vi "20TDewar_Set_Heater_Value.vi"(8 "error in (no error)":errorcluster, 10 "20T-Dewar-Cluster":T1={"Dewar Heater (%)"=0.0, "D-Heater (%) Display"=3.4572, "D-Heater SP"=0.0, "Set D-Heater SP"=FALSE, "Change D-Heater Status"=FALSE, "Dewar Pressure"=0.0, "Dewar heater manual"=FALSE} {"Dewar Pressure" format="%4_5f"; "D-Heater (%) Display" format="%4_5f"; "Dewar Heater (%)" scale=0.0..100.0}, 11 "Mercury Reference In":T2) -> (0 "error out":errorcluster)   [LabVIEW 2016]
uses:
  Equipment/Mercury iXX/Public/Controls/Mercury Reference.ctl
  Equipment/Mercury iXX/Public/Controls/Comms Transport Layer.ctl
  Equipment/Mercury iXX/Private/Controls/Query Dynamic Reference.ctl
  Utility/Monitor Communication/Gustav/20T_Dewar_Cluster.ctl
  Equipment/Mercury iXX/Public/Libraries/Pressure/Open/Open Pressure Device.vi
  Equipment/Mercury iXX/Mercury iXX.lvlib
  Equipment/Mercury iXX/Public/Libraries/Pressure.lvlib
  Equipment/Mercury iXX/Public/Libraries/Control Loop.lvlib
panel:
  # "Dewar Heater (%)"
  # "Dewar Pressure"
  # "Setpoint"
  # "20T Dewar"
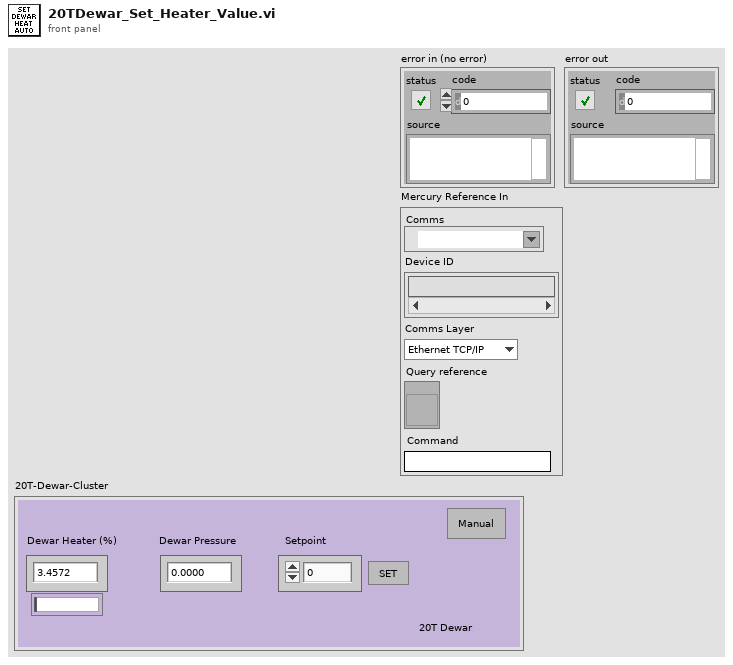
[diagram p1: front panel]
types:
  T1 = typedef "20T_Dewar_Cluster.ctl" = cluster{"Dewar Heater (%)":dbl, "D-Heater (%) Display":dbl, "D-Heater SP":dbl, "Set D-Heater SP":bool, "Change D-Heater Status":bool, "Dewar Pressure":dbl, "Dewar heater manual":bool}
  T2 = typedef "Mercury iXX.lvlib/Mercury Reference.ctl" = cluster{"Comms":refnum<visa-resource-name>, "Device ID":string[], "Comms Layer":T3, "Command":string, "Query reference":T4}
  T3 = typedef "Mercury iXX.lvlib/Comms Transport Layer.ctl" = enum16{"Ethernet TCP/IP", "USB", "ISOBus - RS-232", "GPIB"}
  T4 = typedef "Mercury iXX.lvlib/Query Dynamic Reference.ctl" = refnum<vi>
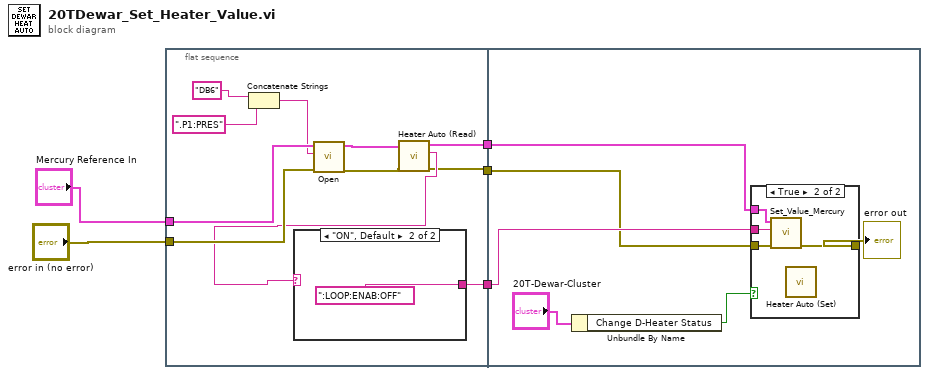
[diagram p0: block diagram]
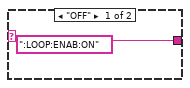
[diagram p2: hidden frame]
diagram:
  n1 = flat-sequence {
    tunnel: "Mercury Reference In" -> [w16]
    tunnel: "error in (no error)" -> [w15]
    tunnel: [w6] -> w3
    tunnel: [w14] -> w2
    tunnel: [w7] -> w1
    tunnel: w3 -> [w19]
    tunnel: w2 -> [w20]
    tunnel: w1 -> [w21]
    frame #0 {
      n2 = Concatenate Strings("DB6", ".P1:PRES" ("Device Identifier")) -> (w11:string)
      n3 = call-poly "Open.vi"("error in (no error)"=w15, "Device Identifier"=w11, "Mercury Reference In"=w16) -> ("error out"=w9:errorcluster, "Mercury Reference Out"=w10:T2)  [unwired: 1 in, 6 out]
      n4 = call "Heater Auto (Read).vi"("error in"=w9, "Mercury Reference In"=w10) -> ("error out"=w6:errorcluster, "Heater Auto"=w8:string, "Mercury Reference Out"=w7:T2)  [unwired: 6 in, 1 out]
      n5 = case shown="\"ON\", Default" w8 {
        tunnel: [":LOOP:ENAB:ON" ("Command") ":LOOP:ENAB:OFF" ("Command")] -> w14
        frame "OFF" {
        }
        frame "ON", Default {
        }
      }
    }
    frame #1 {
      n6 = Unbundle By Name("20T-Dewar-Cluster") -> ("Change D-Heater Status"=w23:bool)
      n7 = case shown="True" w23 {
        tunnel: w19 -> [w25 w26]
        tunnel: [w25 w29] -> w24
        tunnel: w21 -> [_ w28]
        tunnel: w20 -> [_ w27]
        frame False {
        }
        frame True {
          n8 = call "Set_Value_Mercury.vi"("error in"=w26, "Noun(s)"=w27, "Mercury Reference In"=w28) -> ("error out"=w29:errorcluster)  [unwired: 7 in, 1 out]
          n9 = call "Heater Auto (Set).vi"() -> ()  [unwired: 8 in, 4 out]
        }
      }
      "error out" <- w24
    }
  }
